vi "Load_Zspec_Grid_Param_SubVi.vi"(10 "STS Param List":u16, 11 "data\n\n in":T1(array[cluster])) -> (3 "Name":string)   [LabVIEW 2014]
uses:
  <userlib>/Nanonis Prog Interface V5/Nanonis Prog Interface.lvlib
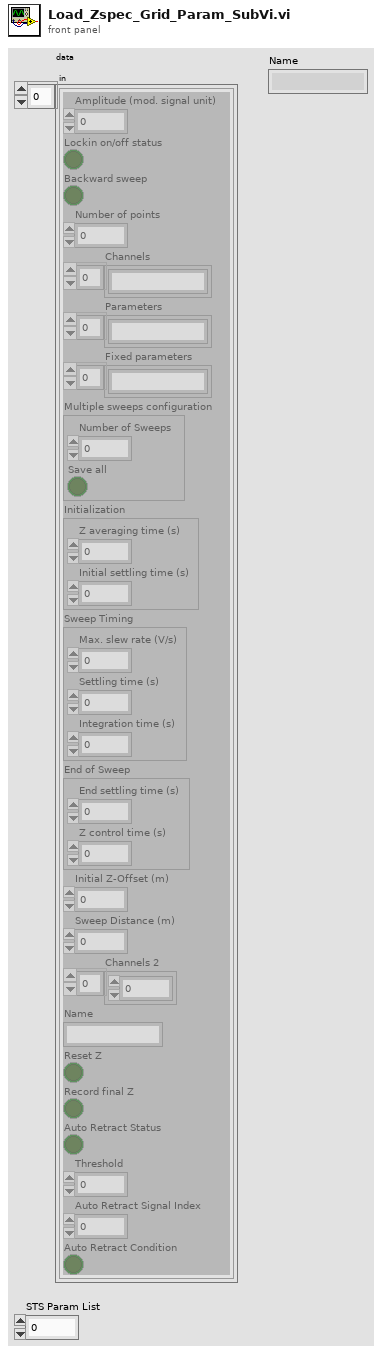
[diagram p1: front panel]
types:
  T1 = cluster{"Amplitude (mod. signal unit)":sgl, "Lockin on/off status":bool, "Backward sweep":bool, "Number of points":i32, "Channels":string[], "Parameters":string[], "Fixed parameters":string[], "Multiple sweeps configuration":cluster{"Number of Sweeps":i32, "Save all":bool}, "Initialization":cluster{"Z averaging time (s)":sgl, "Initial settling time (s)":sgl}, "Sweep Timing":cluster{"Max. slew rate (V/s)":sgl, "Settling time (s)":sgl, "Integration time (s)":sgl}, "End of Sweep":cluster{"End settling time (s)":sgl, "Z control time (s)":sgl}, "Initial Z-Offset (m)":sgl, "Sweep Distance (m)":sgl, "Channels 2":i32[], "Name":string, "Reset Z":bool, "Record final Z":bool, "Auto Retract Status":bool, "Threshold":sgl, "Auto Retract Signal Index":i32, "Auto Retract Condition":bool}[]
  T2 = cluster{"Amplitude (mod. signal unit)":sgl, "Lockin on/off status":bool, "Backward sweep":bool, "Number of points":i32, "Channels":string[], "Parameters":string[], "Fixed parameters":string[], "Multiple sweeps configuration":cluster{"Number of Sweeps":i32, "Save all":bool}, "Initialization":cluster{"Z averaging time (s)":sgl, "Initial settling time (s)":sgl}, "Sweep Timing":cluster{"Max. slew rate (V/s)":sgl, "Settling time (s)":sgl, "Integration time (s)":sgl}, "End of Sweep":cluster{"End settling time (s)":sgl, "Z control time (s)":sgl}, "Initial Z-Offset (m)":sgl, "Sweep Distance (m)":sgl, "Channels 2":i32[], "Name":string, "Reset Z":bool, "Record final Z":bool, "Auto Retract Status":bool, "Threshold":sgl, "Auto Retract Signal Index":i32, "Auto Retract Condition":bool}
  T3 = cluster{"Z averaging time (s)":sgl, "Initial settling time (s)":sgl}
  T4 = cluster{"Max. slew rate (V/s)":sgl, "Settling time (s)":sgl, "Integration time (s)":sgl}
  T5 = cluster{"End settling time (s)":sgl, "Z control time (s)":sgl}
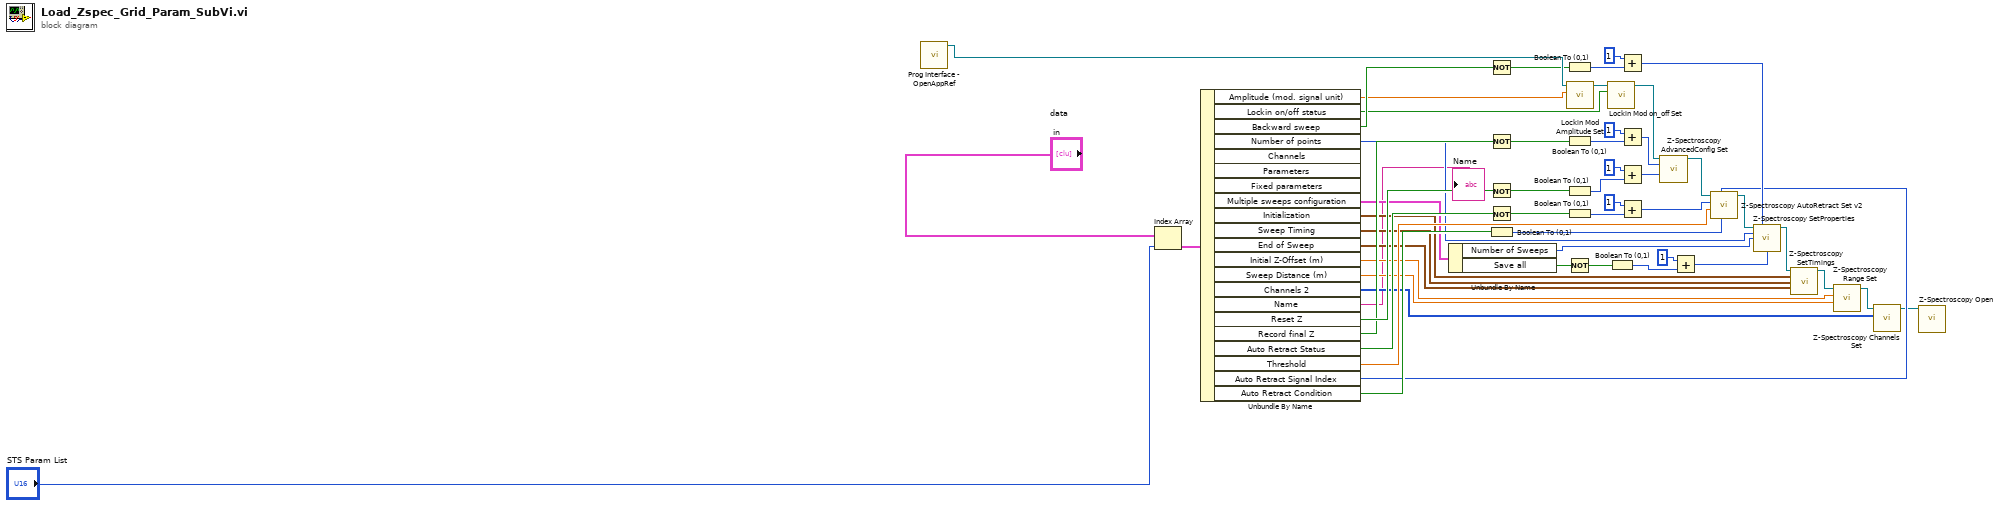
[diagram p0: block diagram]
diagram:
  n1 = call <userlib>:"Prog Interface - OpenAppRef.vi"() -> ("Application reference"=w51:refnum<vi>)  [unwired: 6 in, 1 out]
  n2 = Index Array(array="data\n\n in", index="STS Param List") -> (element=w20:T2)
  n3 = Unbundle By Name(w20) -> ("Amplitude (mod. signal unit)"=w7:sgl, "Lockin on/off status"=w6:bool, "Backward sweep"=w32:bool, "Number of points"=w19:i32, "Multiple sweeps configuration"=w13:cluster{"Number of Sweeps":i32, "Save all":bool}, "Initialization"=w10:T3, "Sweep Timing"=w9:T4, "End of Sweep"=w8:T5, "Initial Z-Offset (m)"=w16:sgl, "Sweep Distance (m)"=w15:sgl, "Channels 2"=w11:i32[], "Name"=→"Name":string, "Reset Z"=w46:bool, "Record final Z"=w43:bool, "Auto Retract Status"=w24:bool, "Threshold"=w28:sgl, "Auto Retract Signal Index"=w21:i32, "Auto Retract Condition"=w26:bool)  [unwired: 3 out]
  n4 = Unbundle By Name(w13) -> ("Number of Sweeps"=w50:i32, "Save all"=w14:bool)
  n5 = Not(x=w32) -> (.not. x?=w31:bool)
  n6 = Not(x=w43) -> (.not. x?=w40:bool)
  n7 = Not(x=w46) -> (.not. x?=w45:bool)
  n8 = Not(x=w24) -> (.not. x?=w23:bool)
  n9 = Boolean To (0,1)(Boolean=w26) -> (0, 1=w27:i16)
  n10 = Boolean To (0,1)(Boolean=w31) -> (0, 1=w30:i16)
  n11 = Boolean To (0,1)(Boolean=w40) -> (0, 1=w39:i16)
  n12 = Boolean To (0,1)(Boolean=w45) -> (0, 1=w44:i16)
  n13 = Boolean To (0,1)(Boolean=w23) -> (0, 1=w22:i16)
  n14 = Not(x=w14) -> (.not. x?=w4:bool)
  n15 = call <userlib>:"Lockin Mod Amplitude Set.vi"("Amplitude (mod. signal unit)"=w7, "Application ref in"=w51) -> ("Application ref out"=w1:refnum<vi>)  [unwired: 8 in, 1 out]
  n16 = call <userlib>:"Lockin Mod on_off Set.vi"("Lockin ON/OFF"=w6, "Application ref in"=w1) -> ("Application ref out"=w38:refnum<vi>)  [unwired: 8 in, 1 out]
  n17 = Boolean To (0,1)(Boolean=w4) -> (0, 1=w2:i16)
  n18 = Add(x=i16 1, y=w30) -> (x+y=w34:i16)
  n19 = Add(x=i16 1, y=w39) -> (x+y=w41:i16)
  n20 = Add(x=i16 1, y=w44) -> (x+y=w48:i16)
  n21 = Add(x=i16 1, y=w22) -> (x+y=w25:i16)
  n22 = call <userlib>:"Z-Spectroscopy AdvancedConfig Set.vi"("Application ref in"=w38, "Record final Z position at the end of the sweep"=w41, "Reset Z at the end of the sweep"=w48) -> ("Application ref out"=w37:refnum<vi>)  [unwired: 11 in, 1 out]
  n23 = Add(x=i16 1, y=w2) -> (x+y=w49:i16)
  n24 = call <userlib>:"Z-Spectroscopy AutoRetract Set v2.vi"("Retract condition"=w27, "Auto retract signal index (-2=no change)"=w21, "Threshold"=w28, "Auto retract"=w25, "Application ref in"=w37) -> ("Application ref out"=w36:refnum<vi>)  [unwired: 5 in, 1 out]
  n25 = call <userlib>:"Z-Spectroscopy SetProperties.vi"("Application ref in"=w36, "Backward sweep"=w34, "Num points"=w19, "Num sweeps"=w50, "Save all sweeps (no change)"=w49) -> ("Application ref out"=w35:refnum<vi>)  [unwired: 9 in, 1 out]
  n26 = call <userlib>:"Z-Spectroscopy SetTimings.vi"("Application ref in"=w35, "Initialization (NaN)"=w10, "Sweep Timing (NaN)"=w9, "End of Sweep (NaN)"=w8) -> ("Application ref out"=w17:refnum<vi>)  [unwired: 10 in, 1 out]
  n27 = call <userlib>:"Z-Spectroscopy Range Set.vi"("Z distance (m)"=w15, "Z offset (m) (NaN=no change)"=w16, "Application ref in"=w17) -> ("Application ref out"=w18:refnum<vi>)  [unwired: 6 in, 1 out]
  n28 = call <userlib>:"Z-Spectroscopy Channels Set.vi"("Channels"=w11, "Application ref in"=w18) -> ("Application ref out"=w12:refnum<vi>)  [unwired: 8 in, 1 out]
  n29 = call <userlib>:"Z-Spectroscopy Open.vi"("Application ref in"=w12) -> ()  [unwired: 13 in, 2 out]
